vi "write.vi"(8 "data to send":string, 11 "connection data":variant) -> (0 "error out":errorcluster)   [LabVIEW 2011]
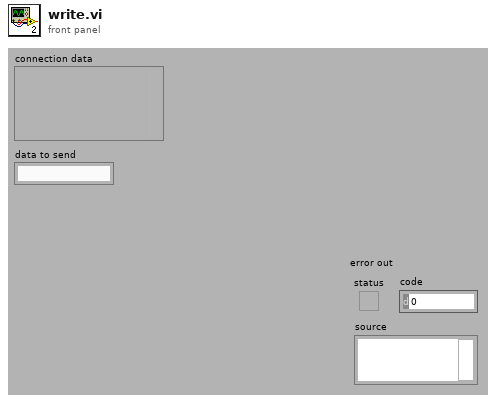
[diagram p1: front panel]
types:
  T1 = enum16{"Channel 1", "Channel 2", "Channel 3", "Real-Time Agent"}
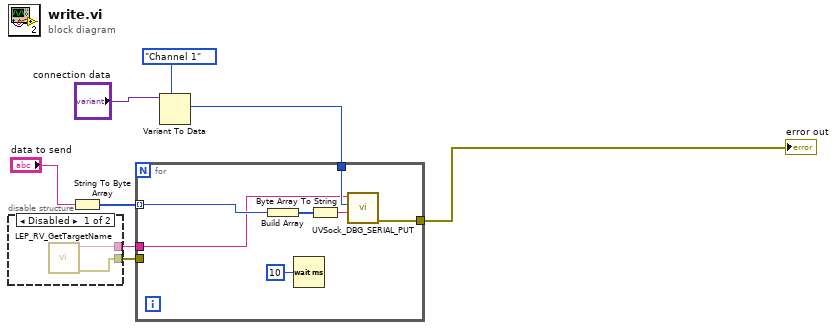
[diagram p0: block diagram]
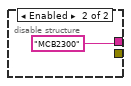
[diagram p2: hidden frame]
diagram:
  n1 = disable-structure shown="Disabled" {
    disable-tunnel: [w9 _] -> w2
    disable-tunnel: [w10 "MCB2300" ("Target Name")] -> w1
    frame Disabled {
      n2 = call "LEP_RV_GetTargetName.vi"() -> ("error out"=w9:errorcluster, "Target Name"=w10:string)  [unwired: 10 in]
    }
    frame Enabled {
    }
  }
  n3 = String To Byte Array(string="data to send") -> (unsigned byte array=w5:u8[])
  n4 = Variant To Data(type=T1."Channel 1" ("Channel"), Variant="connection data") -> (data=w4:T1)  [unwired: 1 in, 1 out]
  n5 = for {
    tunnel: w5 -> [w17] mode=indexing
    tunnel: w4 -> [w13]
    tunnel: [w18] -> w3
    tunnel: w2 -> [_]
    tunnel: w1 -> [w12]
    n6 = Build Array(w17) -> (w16:u8[])
    n7 = Wait (ms)(milliseconds to wait=u32 10) -> ()  [unwired: 1 out]
    n8 = Byte Array To String(unsigned byte array=w16) -> (string=w14:string)
    n9 = call "UVSock_DBG_SERIAL_PUT.vi"("Serial Data"=w14, "Channel"=w13, "Target"=w12) -> ("error out"=w18:errorcluster)  [unwired: 8 in]
  }
  "error out" <- w3
